vi "PH_Stepmotor_BaseClass.contents.vi"   [LabVIEW 2014, in "PH_Stepmotor_BaseClass.lvlib"]
doc: "This class is forseen to control a sixpack (Trinamic Motion Controller).\n\nThis class is part of the PHELIX device layer."
uses:
  PH_Stepmotor_BaseClass.lvlib
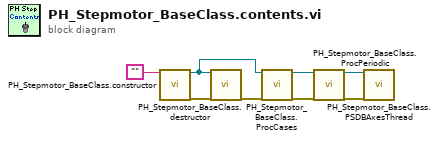
[diagram p0: block diagram]
diagram:
  n1 = call "PH_Stepmotor_BaseClass.constructor.vi"("name"="") -> ("i ref out"=w3:refnum<vi>, "error out"=w5:errorcluster)  [unwired: 16 in, 1 out]
  n2 = call "PH_Stepmotor_BaseClass.destructor.vi"("i ref in"=w3, "error in"=w5) -> ("error out"=w6:errorcluster)  [unwired: 17 in]
  n3 = call "PH_Stepmotor_BaseClass.ProcCases.vi"("i ref in"=w3, "error in"=w6) -> ("i ref out"=w8:refnum<vi>, "error out"=w7:errorcluster)  [unwired: 15 in, 1 out]
  n4 = call "PH_Stepmotor_BaseClass.ProcPeriodic.vi"("i ref in"=w8, "error in"=w7) -> ("i ref out"=w2:refnum<vi>, "error out"=w1:errorcluster)  [unwired: 15 in, 1 out]
  n5 = call "PH_Stepmotor_BaseClass.PSDBAxesThread.vi"("object ref"=w2, "error in (no error)"=w1) -> ()  [unwired: 17 in, 1 out]
